vi "open_relay.vi"(11 "serial_number":string="AB0NXJH7") -> (0 "status":bool, 1 "status_value":u8, 3 "Handle":u64, 4 "message":string)   [LabVIEW 2019]
panel:
  out "status_set_flow_cont":u32(ring) items=["FT_OK", "FT_INVALID_HANDLE", "FT_DEVICE_NOT_FOUND", "FT_DEVICE_NOT_OPENED", "FT_IO_ERROR", "FT_INSUFFICIENT_RESOURCES", "FT_INVALID_PARAMETER", "FT_INVALID_BAUD_RATE", "FT_DEVICE_NOT_OPENED_FOR_ERASE", "FT_DEVICE_NOT_OPENED_FOR_WRITE", "FT_FAILED_TO_WRITE_DEVICE", "FT_EEPROM_READ_FAILED", "FT_EEPROM_WRITE_FAILED", "FT_EEPROM_ERASE_FAILED", "FT_EEPROM_NOT_PRESENT", "FT_EEPROM_NOT_PROGRAMMED", "FT_INVALID_ARGS", "FT_NOT_SUPPORTED", "FT_OTHER_ERROR"]
  out "Pin States":T1
  out "bit_mode":u8 format="%x"
  out "status_set_serial":u32(ring) items=["FT_OK", "FT_INVALID_HANDLE", "FT_DEVICE_NOT_FOUND", "FT_DEVICE_NOT_OPENED", "FT_IO_ERROR", "FT_INSUFFICIENT_RESOURCES", "FT_INVALID_PARAMETER", "FT_INVALID_BAUD_RATE", "FT_DEVICE_NOT_OPENED_FOR_ERASE", "FT_DEVICE_NOT_OPENED_FOR_WRITE", "FT_FAILED_TO_WRITE_DEVICE", "FT_EEPROM_READ_FAILED", "FT_EEPROM_WRITE_FAILED", "FT_EEPROM_ERASE_FAILED", "FT_EEPROM_NOT_PRESENT", "FT_EEPROM_NOT_PROGRAMMED", "FT_INVALID_ARGS", "FT_NOT_SUPPORTED", "FT_OTHER_ERROR"]
  out "status_set_rate":u32(ring) items=["FT_OK", "FT_INVALID_HANDLE", "FT_DEVICE_NOT_FOUND", "FT_DEVICE_NOT_OPENED", "FT_IO_ERROR", "FT_INSUFFICIENT_RESOURCES", "FT_INVALID_PARAMETER", "FT_INVALID_BAUD_RATE", "FT_DEVICE_NOT_OPENED_FOR_ERASE", "FT_DEVICE_NOT_OPENED_FOR_WRITE", "FT_FAILED_TO_WRITE_DEVICE", "FT_EEPROM_READ_FAILED", "FT_EEPROM_WRITE_FAILED", "FT_EEPROM_ERASE_FAILED", "FT_EEPROM_NOT_PRESENT", "FT_EEPROM_NOT_PROGRAMMED", "FT_INVALID_ARGS", "FT_NOT_SUPPORTED", "FT_OTHER_ERROR"]
  in  "Flow Control":u16(ring) items=["None"=0, "RTS-CTS"=256, "DTR-DSR"=512, "XOn-XOff"=1024]
  in  "Parity":u8(ring) items=["FT_PARITY_NONE", "FT_PARITY_ODD", "FT_PARITY_EVEN", "FT_PARITY_MARK", "FT_PARITY_SPACE"]
  in  "Stop Bits":u8(ring) items=["FT_STOP_BITS_1"=0, "FT_STOP_BITS_2"=2]
  in  "Word Length":u8(ring)=8 items=["FT_BITS_7"=7, "FT_BITS_8"=8]
  in  "baud_rate":u32=9600
  # "Default bit mode \n= 0xF0 for FT245R\n= 0x9F for FT232R"
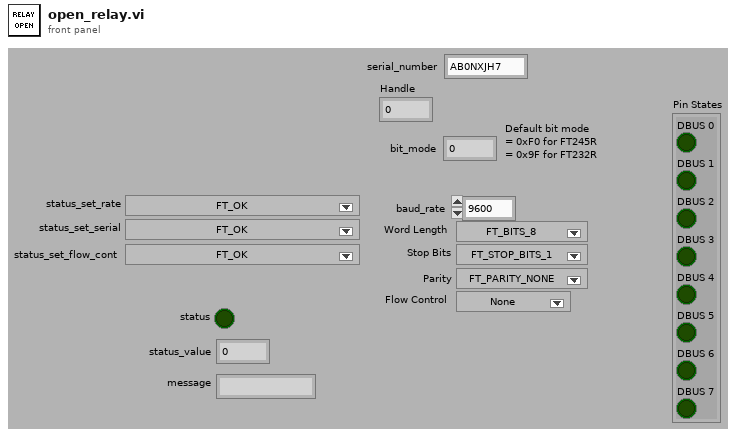
[diagram p1: front panel]
types:
  T1 = cluster{"DBUS 0":bool, "DBUS 1":bool, "DBUS 2":bool, "DBUS 3":bool, "DBUS 4":bool, "DBUS 5":bool, "DBUS 6":bool, "DBUS 7":bool}
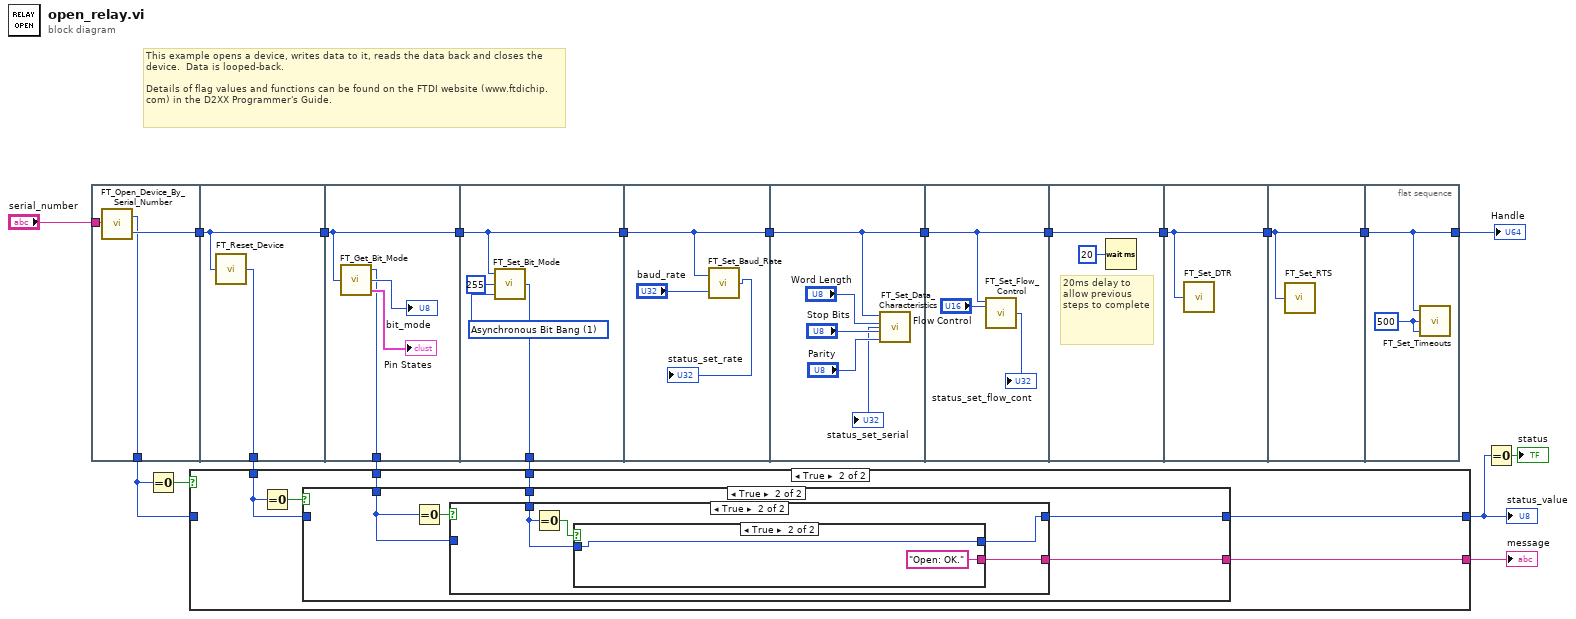
[diagram p0: block diagram]
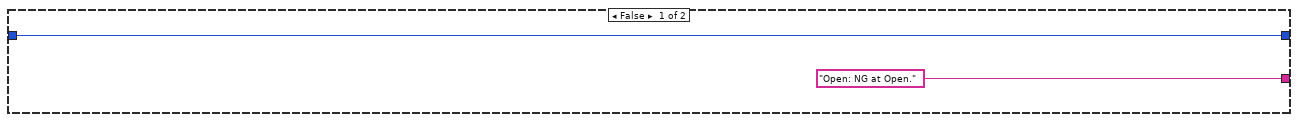
[diagram p2: hidden frame]
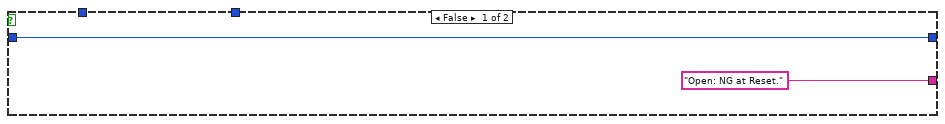
[diagram p3: hidden frame]
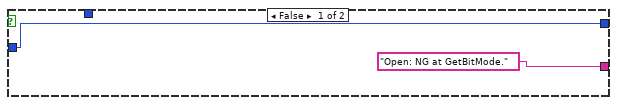
[diagram p4: hidden frame]
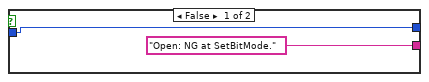
[diagram p5: hidden frame]
diagram:
  # "This example opens a device, writes data to it, reads the data back and closes the device.  Data is looped-back.\n\nDetails of flag values and functions can be found on the FTDI website (www.ftdichip.com) in the D2XX Programmer's Guide."
  n1 = flat-sequence {
    tunnel: [w23] -> w18
    tunnel: "serial_number" -> [w22]
    tunnel: [w21] -> w7
    tunnel: w18 -> [w25]
    tunnel: [w25] -> w15
    tunnel: [w24] -> w5
    tunnel: w15 -> [w29]
    tunnel: [w29] -> w14
    tunnel: [w26] -> w4
    tunnel: w14 -> [w33]
    tunnel: [w33] -> w13
    tunnel: [w30] -> w3
    tunnel: w13 -> [w36]
    tunnel: [w36] -> w16
    tunnel: w16 -> [w41]
    tunnel: [w41] -> w20
    tunnel: w20 -> [w42]
    tunnel: [w42] -> w10
    tunnel: [w45] -> w19
    tunnel: w10 -> [w45]
    tunnel: w19 -> [w47]
    tunnel: [w47] -> w17
    tunnel: w17 -> [w48]
    tunnel: [w48] -> w12
    tunnel: w12 -> [w49]
    tunnel: [w49] -> w9
    frame #0 {
      n2 = call "FT_Open_Device_By_Serial_Number.vi"("Device Serial Number"=w22) -> ("FT_Status"=w21:u32, "Handle"=w23:u64)
    }
    frame #1 {
      n3 = call "FT_Reset_Device.vi"("Handle"=w25) -> ("FT_Status"=w24:u32)
    }
    frame #2 {
      n4 = call "FT_Get_Bit_Mode.vi"("Handle"=w29) -> ("FT_Status"=w26:u32, "Bit Mode"=→"bit_mode":u8, "Pin States"=→"Pin States":T1)
    }
    frame #3 {
      w32 = u8 1 items=["Reset Bit Mode"=0, "Asynchronous Bit Bang"=1, "MPSSE"=2, "Synchronous Bit Bang"=4, "MCU Host Bus Emulation"=8, "Fast Opto-Isolated Serial"=16, "CBUS Bit Bang"=32, "Single Channel 245 Synchronous FIFO"=64] ("Bit Mode")
      n5 = call "FT_Set_Bit_Mode.vi"("Bit Mode"=w32, "Bit Mode Mask"=u8 255, "Handle"=w33) -> ("FT_Status"=w30:u32)
    }
    frame #4 {
      n6 = call "FT_Set_Baud_Rate.vi"("Baud Rate"="baud_rate", "Handle"=w36) -> ("FT_Status"=→"status_set_rate":u32)
    }
    frame #5 {
      n7 = call "FT_Set_Data_Characteristics.vi"("Parity"="Parity", "Stop Bits"="Stop Bits", "Word Length"="Word Length", "Handle"=w41) -> ("FT_Status"=→"status_set_serial":u32)
    }
    frame #6 {
      n8 = call "FT_Set_Flow_Control.vi"("Flow Control"="Flow Control", "Handle"=w42) -> ("FT_Status"=→"status_set_flow_cont":u32)  [unwired: 2 in]
    }
    frame #7 {
      # "20ms delay to allow previous steps to complete"
      n9 = Wait (ms)(milliseconds to wait=u32 20) -> ()  [unwired: 1 out]
    }
    frame #8 {
      n10 = call "FT_Set_DTR.vi"("Handle"=w47) -> ()  [unwired: 1 out]
    }
    frame #9 {
      n11 = call "FT_Set_RTS.vi"("Handle"=w48) -> ()  [unwired: 1 out]
    }
    frame #10 {
      w50 = u32 500 ("Read Timeout")
      n12 = call "FT_Set_Timeouts.vi"("Write Timeout"=w50, "Read Timeout"=w50, "Handle"=w49) -> ()  [unwired: 1 out]
    }
  }
  n13 = Equal To 0?(x=w7) -> (x = 0?=w8:bool)
  n14 = case shown="True" w8 {
    tunnel: [w52 w57] -> w2
    tunnel: w7 -> [w52 _]
    tunnel: ["Open: NG at Open." ("message") w55] -> w6
    tunnel: w5 -> [_ w56]
    tunnel: w4 -> [_ w54]
    tunnel: w3 -> [_ w53]
    frame False {
    }
    frame True {
      n15 = Equal To 0?(x=w56) -> (x = 0?=w58:bool)
      n16 = case shown="True" w58 {
        tunnel: [w60 w64] -> w57
        tunnel: w56 -> [w60 _]
        tunnel: ["Open: NG at Reset." ("message") w62] -> w55
        tunnel: w54 -> [_ w63]
        tunnel: w53 -> [_ w61]
        frame False {
        }
        frame True {
          n17 = Equal To 0?(x=w63) -> (x = 0?=w65:bool)
          n18 = case shown="True" w65 {
            tunnel: [w67 w70] -> w64
            tunnel: w63 -> [w67 _]
            tunnel: ["Open: NG at GetBitMode." ("message") w68] -> w62
            tunnel: w61 -> [_ w69]
            frame False {
            }
            frame True {
              n19 = Equal To 0?(x=w69) -> (x = 0?=w71:bool)
              n20 = case shown="True" w71 {
                tunnel: [w73 w75] -> w70
                tunnel: w69 -> [w73 w75]
                tunnel: ["Open: NG at SetBitMode." ("message") "Open: OK." ("message")] -> w68
                frame False {
                }
                frame True {
                }
              }
            }
          }
        }
      }
    }
  }
  "status_value" <- w2
  "message" <- w6
  n21 = Equal To 0?(x=w2) -> (x = 0?=→"status":bool)
  "Handle" <- w9
